vi "Test Commands.vi"() -> ()   [LabVIEW 2020]
uses:
  _driver/_private/Control/Control Mode.ctl
  _driver/Basic driver/Communication/controls/comm_rate_enum.ctl
  <vilib>/Instr/_visa.llb/VISA Find Search Mode.ctl
  _driver/Chemyx_Syringe_Pump_driver.lvlib
panel:
  in  "Com Port":string(combo)
  in  "Start":bool
  in  "Baud rate":T1
  in  "[x]":T2
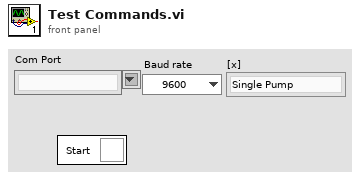
[diagram p1: front panel]
types:
  T1 = typedef "Chemyx_Syringe_Pump_driver.lvlib/comm_rate_enum.ctl" = enum16{"9600", "38400"}
  T2 = typedef "Chemyx_Syringe_Pump_driver.lvlib/Control Mode.ctl" = enum16{"Single Pump", "Pump Channel 1", "Pump Channel 2", "Cycle Mode"}
  T3 = typedef "VISA Find Search Mode.ctl" = u32
  T4 = typedef "Chemyx_Syringe_Pump_driver.lvlib/Pump_status_enum.ctl" = enum16{"Pump Idle", "Pump Running", "Pump Paused", "Pump Delay", "Pump Stalled", "Pump Error"}
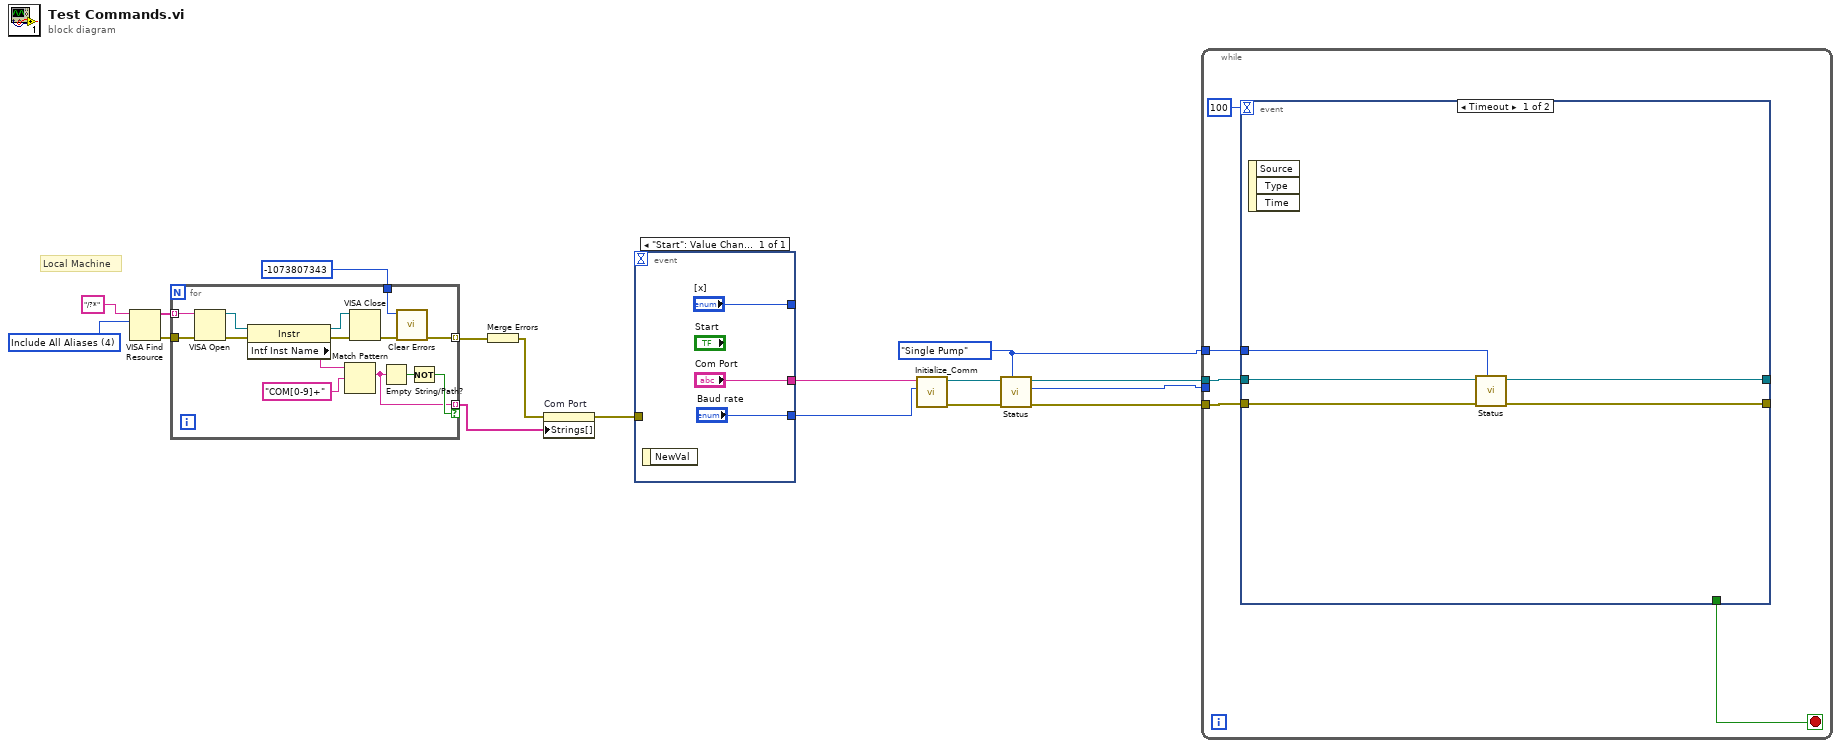
[diagram p0: block diagram]
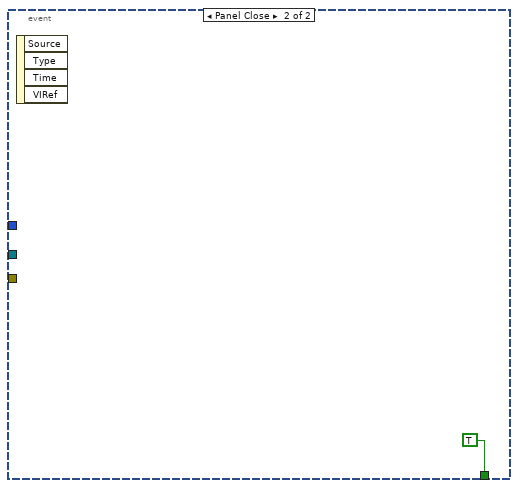
[diagram p2: hidden frame]
diagram:
  w3 = Control_Mode."Single Pump" ("[x]")
  w11 = T3 4 items=["Canonical Names Only"=0, "Aliases Only"=2, "Include Matching Aliases"=3, "Include All Aliases"=4] ("Search Mode")
  # "Local Machine"
  n1 = VISA Find Resource(10:w11, 11:"/?*" ("expression (\"?*\")")) -> (0:w12:errorcluster, 3:w10:string[])  [unwired: 1 in, 1 out]
  n2 = for {
    tunnel: w10 -> [w27] mode=indexing
    tunnel: w12 -> [w25]
    tunnel: [w22] -> w9 mode=indexing
    tunnel: [w19] -> w15 mode=indexing if=w21
    tunnel: -1073807343 ("code") -> [w18]
    n3 = VISA Open(error in (no error)=w25, VISA resource name=w27) -> (VISA resource name=w30:refnum<visa-resource-name>, error out=w28:errorcluster)  [unwired: 3 in]
    n4 = property class="Instr"(reference=w30, error in=w28) -> (reference out=w31:refnum<visa-resource-name>, error out=w29:errorcluster, "Intf Inst Name"=w20:string)
    n5 = Match Pattern(string=w20, regular expression="COM[0-9]+") -> (match substring=w19:string)  [unwired: 1 in, 3 out]
    n6 = VISA Close(VISA resource name=w31, error in (no error)=w29) -> (error out=w23:errorcluster)
    n7 = Empty String/Path?(string/path=w19) -> (empty?=w26:bool)
    n8 = call <vilib>:"Clear Errors.vi"("error in (no error)"=w23, "specific error code to clear (0: all)"=w18) -> ("error out"=w22:errorcluster)  [unwired: 4 in, 1 out]
    n9 = Not(x=w26) -> (.not. x?=w21:bool)
  }
  n10 = Merge Errors(w9) -> (w8:errorcluster)
  n11 = property on="Com Port" class="CmbBox"(error in=w8, "Strings[]"=w15) -> (error out=w7:errorcluster)  [unwired: 1 in, 1 out]
  n12 = event shown="[0] \"Start\": Value Change" {
    selector: _ -> [_]
    dyn-events: _ -> [_]
    timeout: _ -> [_]
    tunnel: ["Com Port"] -> w17
    tunnel: ["Baud rate"] -> w16
    tunnel: w7 -> [_]
    tunnel: ["[x]"] -> _
    event "Start": Value Change {
      n13 = event-data() -> ()  [unwired: 1 in, 1 out]
    }
  }
  n14 = call "Initialize_Comm.vi"("Baud rate"=w16, "Serial Port in"=w17) -> ("error out"=w5:errorcluster, "Serial Port out"=w6:refnum<visa-resource-name>)  [unwired: 8 in]
  n15 = call "Status.vi"("[x]"=w3, "error in (no error)"=w5, "Serial Port in"=w6) -> ("error out"=w1:errorcluster, "Status"=w2:T4, "Serial Port out"=w4:refnum<visa-resource-name>)  [unwired: 6 in]
  n16 = while {
    tunnel: w4 -> [w39]
    tunnel: w3 -> [w36]
    tunnel: w2 -> [_]
    tunnel: w1 -> [w38]
    stop <- w35 stop-if-true
    n17 = event shown="[0] Timeout" {
      selector: _ -> [_ _]
      dyn-events: _ -> [_ _]
      timeout: 100 -> [_ _]
      tunnel: w39 -> [w44 _]
      tunnel: w38 -> [w43 _]
      tunnel: [w42 _] -> _
      tunnel: [w41 _] -> _
      tunnel: w36 -> [w40 _]
      tunnel: [_ TRUE] -> w35
      event Timeout {
        n18 = event-data() -> ()  [unwired: 1 in, 3 out]
        n19 = call "Status.vi"("[x]"=w40, "error in (no error)"=w43, "Serial Port in"=w44) -> ("error out"=w42:errorcluster, "Serial Port out"=w41:refnum<visa-resource-name>)  [unwired: 6 in, 1 out]
      }
      event Panel Close {
        n20 = event-data() -> ()  [unwired: 1 in, 4 out]
      }
    }
  }
